vi "test-diff-centripital-acceleration-constraint.vi"(8 "error in (no error)":errorcluster) -> (0 "error out 2":errorcluster, 3 "Test Passed":bool)   [LabVIEW 2019]
uses:
  <vilib>/Rock Robotics/WPI/ThirdParty/JAS_Junk/TrajLib/POSE2D.ctl
  <vilib>/Rock Robotics/WPI/ThirdParty/JAS_Junk/TrajLib/TRANSLATION2D.ctl
  <vilib>/Rock Robotics/WPI/ThirdParty/JAS_Junk/TrajLib/ROTATION2D.ctl
  <vilib>/Rock Robotics/WPI/ThirdParty/JAS_Junk/TrajLib/CentripetalAccelConstraint_New.vi
  <vilib>/Rock Robotics/WPI/ThirdParty/JAS_Junk/TrajLib/Trajectory_Library.lvlib
panel:
  out "Centrip Accel Limit":dbl
  out "Max Centrip Accel":dbl
  out "XY Graph":cluster{dbl[], dbl[]}[](graph)
  out "Waypoints":T1[](array[typedef]) {"ROTATION"."SIN" format="%13.4f"; "ROTATION"."COS" format="%13.4f"; "ROTATION"."VALUE" format="%13.4f"; "TRANSLATION"."Y" format="%14.3f"; "TRANSLATION"."X" format="%14.3f"}
  out "TotalTImeSecs":dbl
  out "Centrip Accel Exceeded":bool
  out "error out":errorcluster
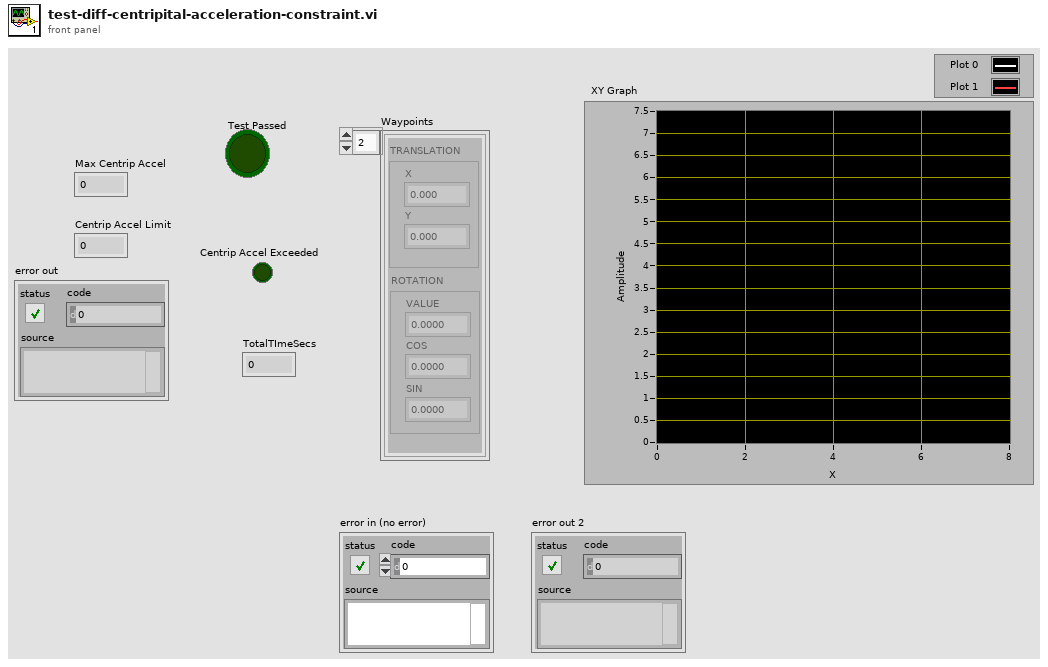
[diagram p1: front panel]
types:
  T1 = typedef "Trajectory_Library.lvlib/POSE2D.ctl" = cluster{"TRANSLATION":T2, "ROTATION":T3}
  T2 = typedef "Trajectory_Library.lvlib/TRANSLATION2D.ctl" = cluster{"X":dbl, "Y":dbl}
  T3 = typedef "Trajectory_Library.lvlib/ROTATION2D.ctl" = cluster{"VALUE":dbl, "COS":dbl, "SIN":dbl}
  T4 = typedef "Trajectory_Library.lvlib/TRAJ_CONFIG.ctl" = cluster{"MaxVelocity":dbl, "Max Acceleration":dbl, "StartVelocity":dbl, "End Velocity":dbl, "Reversed":bool, "DiffDrKineConstntDefined":bool, "CentAcellConstntDefined":bool, "DiffDrVoltConstntDefined":bool, "DIFF_DRIVE_KINE_CONSTRAINT":T5, "CENTRIPETAL_ACCEL_CONSTRAINT":T7, "SwerveDrKineConstntDefined":bool, "SWERVE_DRIVE_KINE_CONSTRAINT":T8, "DIFF_DRIVE_VOLTAGE_CONSTRAINT":T11, "MECANUM_DRIVE_KINE_CONSTRAINT":T13, "MecanumDrKineConstntDefined":bool}
  T5 = typedef "Trajectory_Library.lvlib/TRAJ_CONSTRAINT_DIIF_DRIVE_KINEMATICS.ctl" = cluster{"Max Speed (M/S)":dbl, "DIFF_DRIVE_KINEMATICS":T6, "Max Accel (M/S2)":dbl}
  T6 = typedef "Trajectory_Library.lvlib/DIFF_DRIVE_KINEMATICS.ctl" = cluster{"TrackWidth_Meters":dbl}
  T7 = typedef "Trajectory_Library.lvlib/TRAJ_CONSTRAINT_CENTRIPETAL_ACCEL.ctl" = cluster{"Max Cent Accel":dbl}
  T8 = typedef "Trajectory_Library.lvlib/TRAJ_CONSTRAINT_SWERVE_DRIVE_KINEMATICS.ctl" = cluster{"Max Speed (M/S)":dbl, "SwerveKinematics":T9}
  T9 = typedef "Trajectory_Library.lvlib/SWERVE_DRIVE_KINEMATICS.ctl" = cluster{"NumModules":i32, "InverseKinematics":T10, "ForwardKinematics":T10, "Modules":T2[], "PrevCoR":T2}
  T10 = typedef "NI_Matrix.lvlib/RealMatrix.ctl" = dbl[][]
  T11 = typedef "Trajectory_Library.lvlib/TRAJ_CONSTRAINT_DIIF_DRIVE_VOLTAGE.ctl" = cluster{"Max Voltage":dbl, "DIFF_DRIVE_KINEMATICS":T6, "SIMPLE_MOTOR_FF":T12}
  T12 = typedef "Trajectory_Library.lvlib/SIMPLE_MOTOR_FF.ctl" = cluster{"Ks":dbl, "Kv":dbl, "Ka":dbl}
  T13 = typedef "Trajectory_Library.lvlib/TRAJ_CONSTRAINT_MECA_DRIVE_KINEMATICS.ctl" = cluster{"Max Speed (M/S)":dbl, "MECA_DRIVE_KINEMATICS":T14}
  T14 = typedef "Trajectory_Library.lvlib/MECA_DRIVE_KINEMATICS.ctl" = cluster{"FrontLeft":T2, "FrontRight":T2, "RearLeft":T2, "RearRight":T2, "InverseKinematics":T10, "ForwardKinematics":T10, "PrevCoR":T2}
  T15 = typedef "Trajectory_Library.lvlib/TRAJECTORY.ctl" = cluster{"TotalTImeSecs":dbl, "States":T16[]}
  T16 = typedef "Trajectory_Library.lvlib/TRAJ_STATE.ctl" = cluster{"TimeSeconds":dbl, "Velocity":dbl, "Acceleration":dbl, "POSE":T1, "Curvature":dbl}
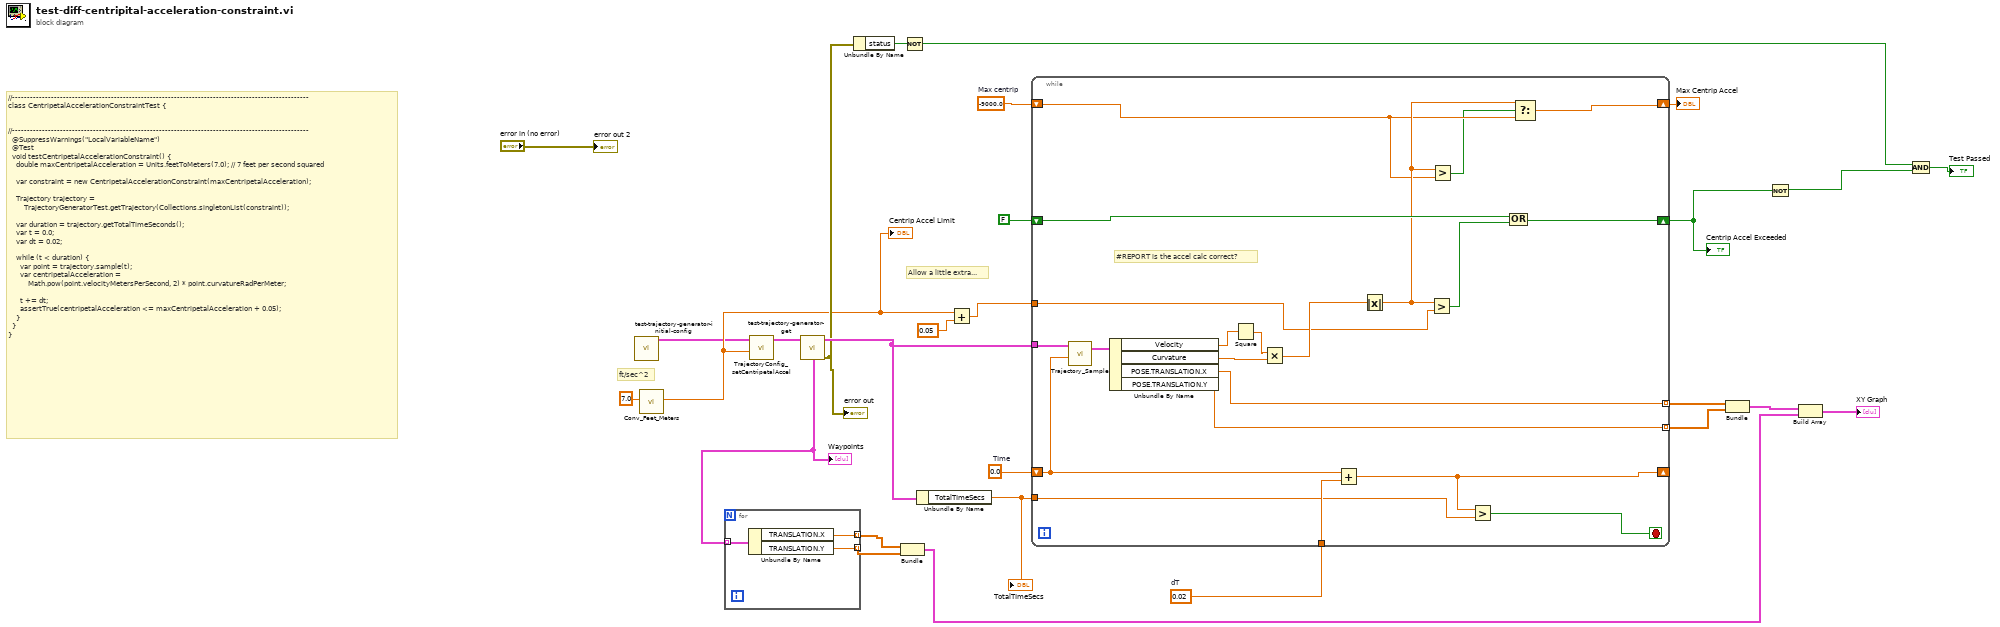
[diagram p0: block diagram]
diagram:
  w12 = -9000.0  # Max centrip
  w25 = 0.02  # dT
  w27 = 0.0  # TIme
  # "ft/sec^2"
  # "//---------------------------------------------------------------------------------------------------\nclass CentripetalAccelerationConstraintTest {\n\n\n//---------------------------------------------------------------------------------------------------\n  @SuppressWarnings(\"LocalVariableName\")\n  @Test\n  void testCentripetalAccelerationConstraint() {\n    double maxCentripetalAcceleration = Units.feetToMeters(7.0); // 7 feet per second squared\n\n    var constraint = new CentripetalAccelerationConstraint(maxCentripetalAcceleration);\n\n    Trajectory trajectory =\n        TrajectoryGeneratorTest.getTrajectory(Collections.singletonList(constraint));\n\n    var duration = trajectory.getTotalTimeSeconds();\n    var t = 0.0;\n    var dt = 0.02;\n\n    while (t < duration) {\n      var point = trajectory.sample(t);\n      var centripetalAcceleration =\n          Math.pow(point.velocityMetersPerSecond, 2) * point.curvatureRadPerMeter;\n\n      t += dt;\n      assertTrue(centripetalAcceleration <= maxCentripetalAcceleration + 0.05);\n    }\n  }\n}"
  # "Allow a little extra..."
  n1 = call "test-trajectory-generator-initial-config.vi"() -> ("traj_config"=w2:T4)  [unwired: 11 in]
  n2 = call <vilib>:"Conv_Feet_Meters.vi"("Feet"=7.0) -> ("Meters"=w3:dbl)  [unwired: 10 in]
  "Centrip Accel Limit" <- w3
  n3 = call <vilib>:"TrajectoryConfig_setCentripetalAccel.vi"("Max Cent Accel"=w3, "inTRAJECTORY_CONFIG"=w2) -> ("outTRAJECTORY_CONFIG"=w28:T4)  [unwired: 9 in]
  n4 = call "test-trajectory-generator-get.vi"("traj_config"=w28) -> ("error out"=w7:errorcluster, "TRAJECTORY"=w24:T15, "Waypoints"=w20:T1[])  [unwired: 8 in]
  "error out" <- w7
  "Waypoints" <- w20
  n5 = for {
    tunnel: w20 -> [w31] mode=indexing
    tunnel: [w30] -> w19 mode=indexing
    tunnel: [w29] -> w18 mode=indexing
    n6 = Unbundle By Name(w31) -> ("TRANSLATION.X"=w30:dbl, "TRANSLATION.Y"=w29:dbl)
  }
  n7 = Unbundle By Name(w7) -> ("status"=w6:bool)
  n8 = Bundle(w19, w18) -> (w14:cluster{dbl[], dbl[]})  [unwired: 1 in]
  n9 = Not(x=w6) -> (.not. x?=w5:bool)
  n10 = Unbundle By Name(w24) -> ("TotalTImeSecs"=w26:dbl)
  "TotalTImeSecs" <- w26
  n11 = Add(x=w3, y=0.05) -> (x+y=w22:dbl)
  n12 = while {
    tunnel: w26 -> [w50]
    shift-right: [w51] -> _
    shift-left: w27 -> [w47]
    tunnel: w25 -> [w52]
    tunnel: w24 -> [w48]
    shift-right: [w43] -> w8
    shift-left: FALSE -> [w44]
    tunnel: w22 -> [w32]
    tunnel: [w41] -> w17 mode=indexing
    tunnel: [w40] -> w16 mode=indexing
    shift-right: [w39] -> w11
    shift-left: w12 -> [w37]
    stop <- w49 stop-if-true
    # "#REPORT is the accel calc correct?"
    n13 = call <vilib>:"Trajectory_Sample.vi"("Time"=w47, "InputTRAJECTORY"=w48) -> ("OutputTRAJ_STATE"=w46:T16)  [unwired: 9 in]
    n14 = Unbundle By Name(w46) -> ("Velocity"=w35:dbl, "Curvature"=w45:dbl, "POSE.TRANSLATION.X"=w41:dbl, "POSE.TRANSLATION.Y"=w40:dbl)
    n15 = Square(x=w35) -> (x^2=w34:dbl)
    n16 = Multiply(x=w34, y=w45) -> (x*y=w33:dbl)
    n17 = Add(x=w47, y=w52) -> (x+y=w51:dbl)
    n18 = Absolute Value(x=w33) -> (abs(x)=w38:dbl)
    n19 = Greater?(x=w38, y=w32) -> (0:w42:bool)
    n20 = Greater?(x=w38, y=w37) -> (0:w36:bool)
    n21 = Greater?(x=w51, y=w50) -> (0:w49:bool)
    n22 = Compound Arithmetic op=OR(w44, w42) -> (w43:bool)
    n23 = Select(t=w38, s=w36, f=w37) -> (s? t:f=w39:dbl)
  }
  "Centrip Accel Exceeded" <- w8
  "Max Centrip Accel" <- w11
  n24 = Bundle(w17, w16) -> (w15:cluster{dbl[], dbl[]})  [unwired: 1 in]
  n25 = Not(x=w8) -> (.not. x?=w9:bool)
  n26 = Build Array(w15, w14) -> (→"XY Graph":cluster{dbl[], dbl[]}[])
  n27 = Compound Arithmetic op=AND(w5, w9) -> (→"Test Passed":bool)
  "error out 2" <- "error in (no error)"
